vi "Display_Recipe.vi"(0 "Recipes":string[][](array[string])=[["1", "Rice", "66PL10", "12PL3", "10PL4"], ["2", "Frozen Dinner", "5PL8", "10PL2", ""], ["3", "Popcorn", "5PL3", "", ""]], 1 "State In":T1, 5 "Recipe":i32, 7 "Step In":i32, 9 "Time Remaining In":dbl, 11 "error in (no error)":errorcluster) -> (3 "State Out":T1=enum."Staged", 4 "Display Out":string, 6 "Target Time":dbl, 8 "Step Out":i32, 10 "Time Remaining Out":dbl, 15 "error out":errorcluster)   [LabVIEW 2026]
uses:
  controls/System_Status.ctl
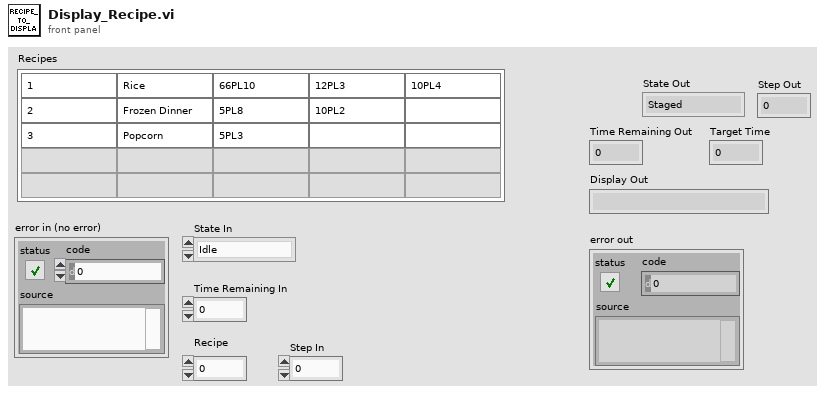
[diagram p1: front panel]
types:
  T1 = typedef "System_Status.ctl" = enum16{"Idle", "Staged", "Cooking", "Paused", "Buzzer Alert"}
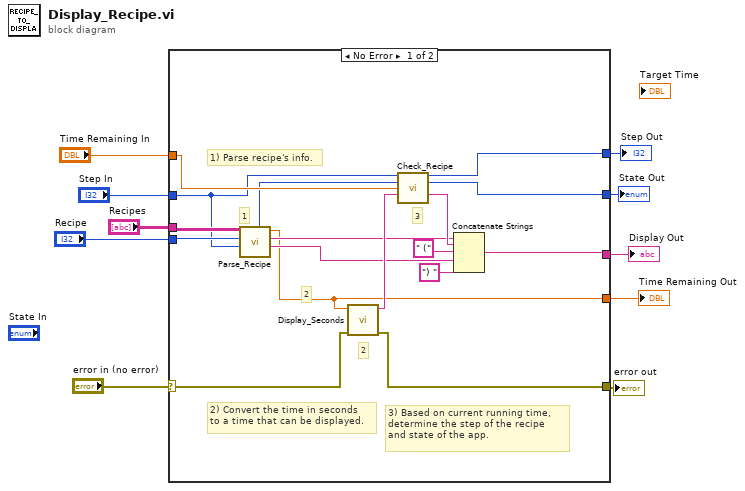
[diagram p0: block diagram]
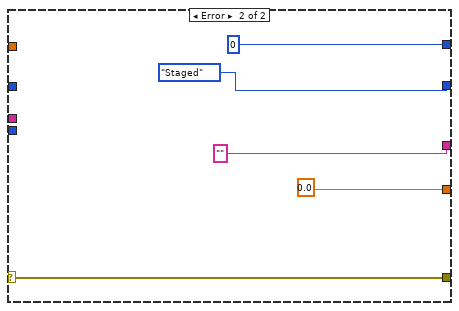
[diagram p2: hidden frame]
diagram:
  n1 = case shown="No Error" "error in (no error)" {
    selector: "error in (no error)" -> [w24 w32]
    tunnel: "Recipes" -> [w17 _]
    tunnel: [w23 w32] -> w9
    tunnel: [w25 ""] -> w8
    tunnel: "Step In" -> [w12 _]
    tunnel: "Recipe" -> [w16 _]
    tunnel: [w11 0.0] -> w4
    tunnel: "Time Remaining In" -> [w20 _]
    tunnel: [w22 0] -> w1
    tunnel: [w21 System_Status."Staged" ("State")] -> w2
    frame No Error {
      # "3) Based on current running time, \ndetermine the step of the recipe\nand state of the app."
      # "3"
      # "2) Convert the time in seconds \nto a time that can be displayed."
      # "2"
      # "2"
      # "1"
      # "1) Parse recipe's info."
      n2 = call "Parse_Recipe.vi"("Step In"=w12, "Recipe"=w16, "Recipes"=w17) -> ("PL"=w13:string, "Food"=w14:string, "Time Remaining"=w11:dbl, "Number of Steps"=w15:i32)  [unwired: 4 in, 1 out]
      n3 = call "Display_Seconds.vi"("error in (no error)"=w24, "Time (s) In"=w11) -> ("error out"=w23:errorcluster, "Display Out"=w18:string)  [unwired: 7 in, 1 out]
      n4 = call "Check_Recipe.vi"("Step In"=w12, "Number of Steps"=w15, "Time Remaining"=w20, "Display In"=w18) -> ("Step Out"=w22:i32, "State"=w21:T1, "Display Out"=w19:string)  [unwired: 8 in, 1 out]
      n5 = Concatenate Strings(w14, w19, " (", w13, ") ") -> (w25:string)
    }
    frame Error {
    }
  }
  "error out" <- w9
  "Display Out" <- w8
  "Time Remaining Out" <- w4
  "State Out" <- w2
  "Step Out" <- w1
